vi "ma_Find First Error.vi"(4 "error array in":errorcluster[](array[cluster]), 5 "error in 3 (no error)":errorcluster, 6 "error in 2 (no error)":errorcluster, 7 "error in 1 (no error)":errorcluster) -> (0 "error out":errorcluster)   [LabVIEW 2020, in "NI_MABase.lvlib"]
doc: "Merges error I/O clusters from different functions."
uses:
  NI_MABase.lvlib
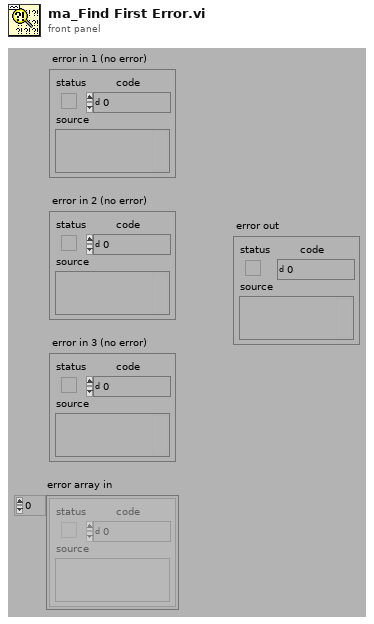
[diagram p1: front panel]
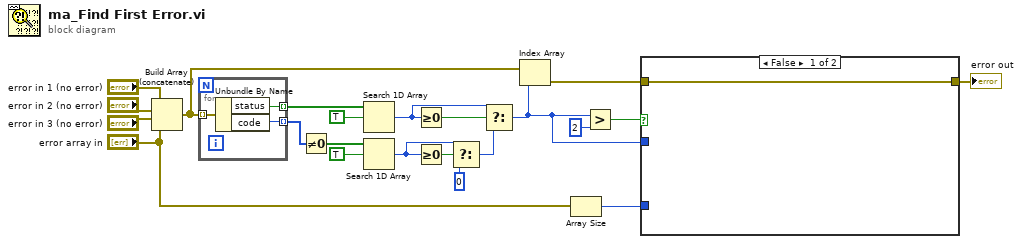
[diagram p0: block diagram]
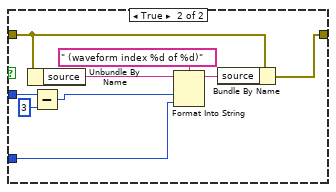
[diagram p2: hidden frame]
diagram:
  n1 = Build Array (concatenate)("error in 1 (no error)", "error in 2 (no error)", "error in 3 (no error)", "error array in") -> (w10:errorcluster[])
  n2 = for {
    tunnel: w10 -> [w25] mode=indexing
    tunnel: [w24] -> w19 mode=indexing
    tunnel: [w23] -> w16 mode=indexing
    n3 = Unbundle By Name(w25) -> ("status"=w24:bool, "code"=w23:i32)
  }
  n4 = Not Equal To 0?(x=w16) -> (x != 0?=w8:bool[])
  n5 = Search 1D Array(1D array=w19, element=TRUE) -> (index of element=w11:i32)  [unwired: 1 in]
  n6 = Search 1D Array(1D array=w8, element=TRUE) -> (index of element=w15:i32)  [unwired: 1 in]
  n7 = Greater Or Equal To 0?(x=w11) -> (x >= 0?=w12:bool)
  n8 = Greater Or Equal To 0?(x=w15) -> (x >= 0?=w14:bool)
  n9 = Select(t=w15, s=w14, f=0) -> (s? t:f=w13:i32)
  n10 = Select(t=w11, s=w12, f=w13) -> (s? t:f=w3:i32)
  n11 = Index Array(array=w10, index=w3) -> (element=w6:errorcluster)
  n12 = Array Size(array="error array in") -> (size(s)=w1:i32)
  n13 = Greater?(x=w3, y=2) -> (0:w4:bool)
  n14 = case shown="False" w4 {
    tunnel: w6 -> [w26 w31]
    tunnel: [w26 w30] -> w5
    tunnel: w3 -> [_ w35]
    tunnel: w1 -> [_ w32]
    frame False {
    }
    frame True {
      n15 = Unbundle By Name(w31) -> ("source"=w28:string)
      n16 = Subtract(x=w35, y=3) -> (x-y=w33:i32)
      n17 = Format Into String(format string=" (waveform index %d of %d)" ("initial string"), initial string=w28, w33, w32) -> (resulting string=w27:string)  [unwired: 1 in, 1 out]
      n18 = Bundle By Name(cluster=w31, "source"=w27) -> (w30:errorcluster)
    }
  }
  "error out" <- w5
